vi "DB UI - Transaction Details.vi"(7 "DB Connection":T4={"Open"=TRUE, "Close"=TRUE}, 8 "error in (no error)":errorcluster, 10 "Transaction":T5, 11 "connection reference 2":T2) -> (0 "SUMMARY":errorcluster, 3 "connection reference":T2)   [LabVIEW 2013]
uses:
  <vilib>/addons/database/Connection.llb/Conn ObjectReference.ctl
  Controls/DB - OpenClose.ctl
  Controls/Transaction Cluster.ctl
  Controls/Debug Tab.ctl
  <vilib>/Utility/miscctls.llb/LVPointTypeDef.ctl
  <vilib>/addons/database/Connection.llb/Conn Execute.vi
  <vilib>/addons/database/Recordset.llb/Rec Fetch Recordset Data (R).vi
  <vilib>/addons/database/Recordset.llb/Rec Destroy - Connection.vi
  Controls/Global SRTRS.vi
  <vilib>/addons/database/Connection.llb/DB Tools Open Connec (String).vi
  <vilib>/addons/database/_DB Variant To Data/Database Variant To Data.xnode
  <vilib>/addons/database/NI_Database_API.lvlib
panel:
  in  "Tab Control":T1
  out "Connection Information":T3={"Connection "="SQL Server 32bit HPEnvy", "Username"="admin", "Password"="admin123"}
  in  "DB.Schema.Table\nSRTRS.Execute.Header":string="SRTRS.Execute.Header"
  in  "DB.Schema.Table \nSRTRS.Config.Plant":string="SRTRS.Config.Plant"
  out "data":string[](array[string])
  out "SQL Statement":string
  in  "DB.Schema.Table \nSRTRS.Config.Station":string="SRTRS.Config.Station"
  in  "DB.Schema.Table \nSRTRS.Execute.TransactionResult":string="SRTRS.Execute.TransactionResult"
  in  "DB.Schema.Table \nSRTRS.Config.System":string="SRTRS.Config.System"
  out "Close 2":errorcluster
  in  "Details [CaptionOnly]":string caption="Details"
  in  "Header [CaptionOnly]":string caption="Header"
  in  "Close":bool caption="Setup Save"
  out "[PerformedOn]":string caption="Performed On"
  out "[LastSavedOn]":string caption="Last Saved On"
  out "[LastSavedBy]":string caption="Last Saved By"
  out "Station [Description]":string caption="Station"
  out "System [Description]":string caption="System"
  out "Plant [Description]":string caption="Plant"
  out "[StationId]":string caption="Station"
  out "[SystemId]":string caption="System"
  out "[PlantId]":string caption="Plant"
  out "[TransactionRunNo]":string caption="Run No."
  out "[TransactionNo]":string caption="Transaction No."
  # "2014-10-28 13:44\nh.[PlantId]                          ,p.[Description]           ,h.[StationId]                  ,st.[Description]             ,sy.[SystemId]                ,sy.[Description]           ,h.[LastSavedBy]           ,h.[LastSavedOn]          ,t.[PerformedOn]"
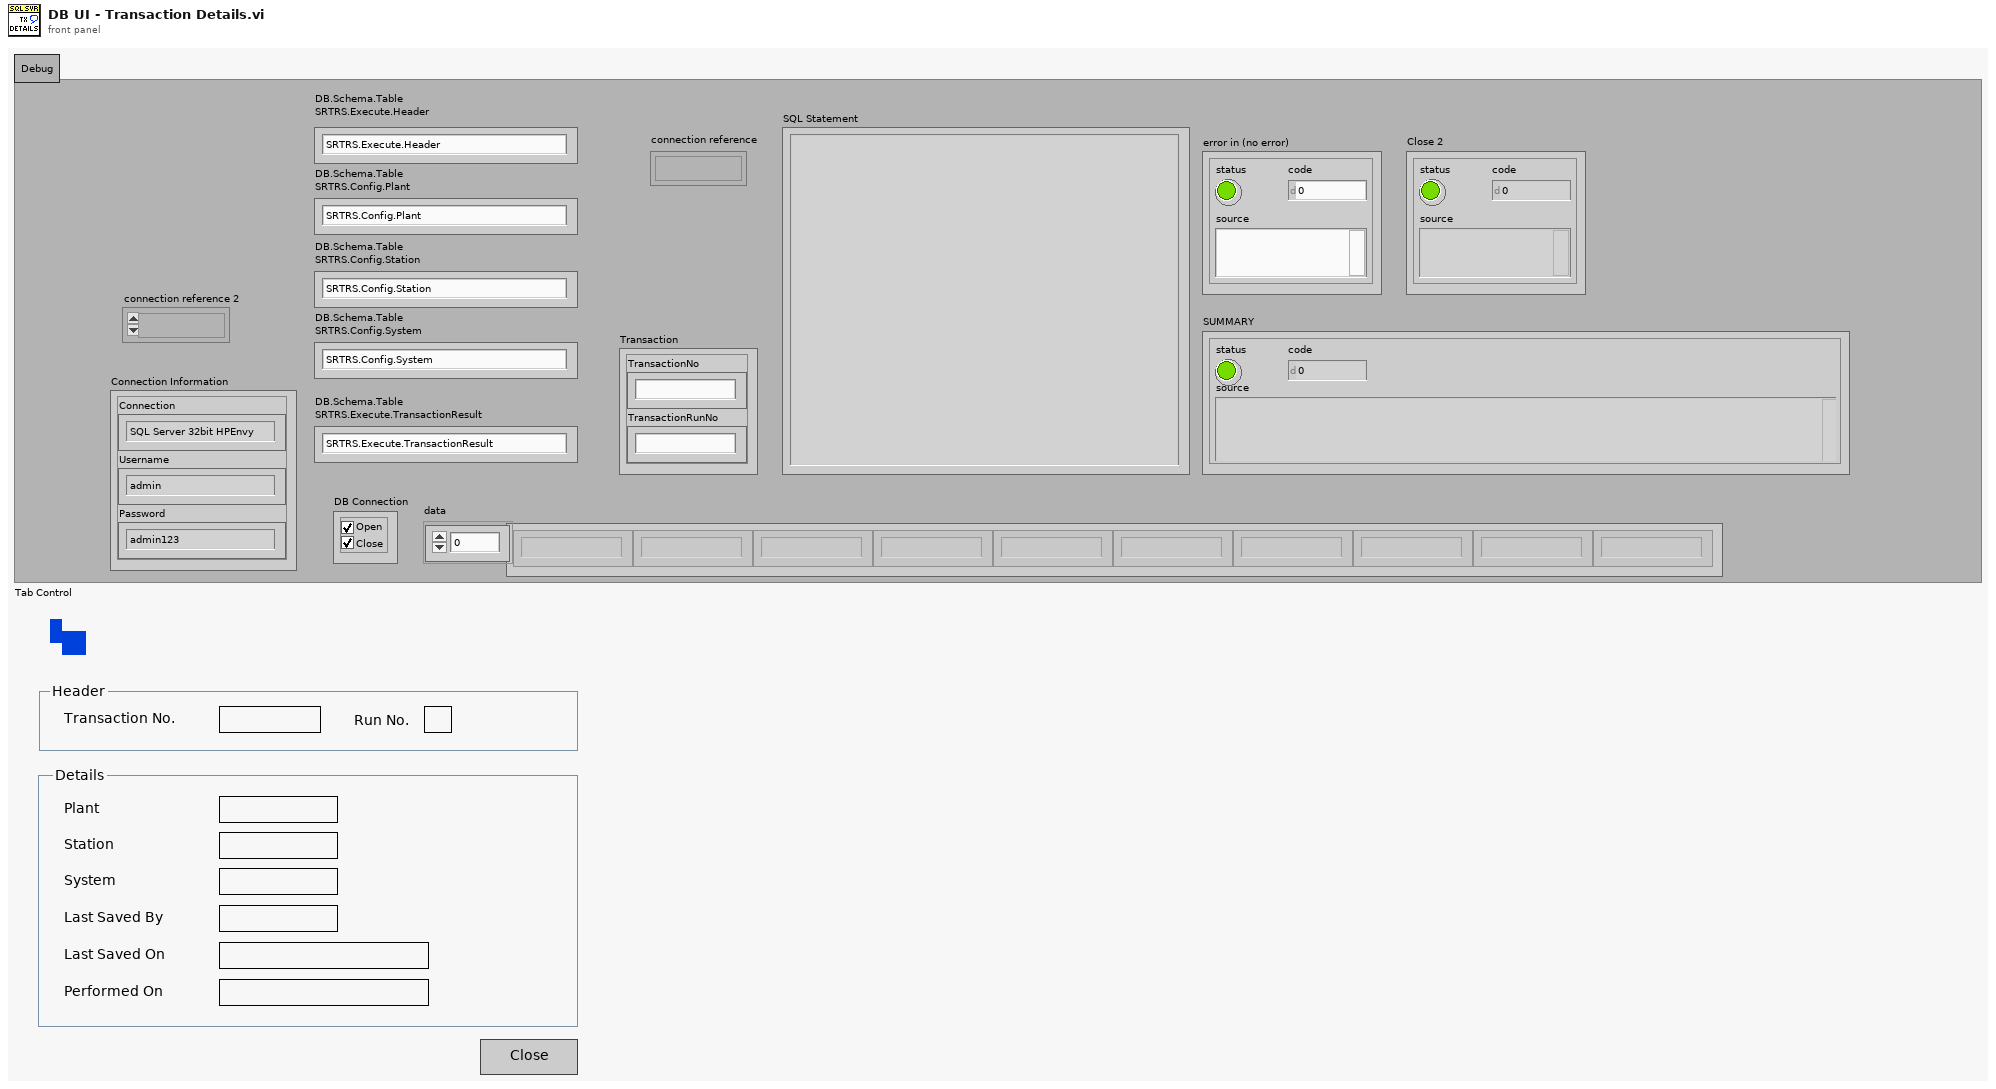
[diagram p1: front panel]
types:
  T1 = typedef "Debug Tab.ctl" = enum32{"Debug"}
  T2 = typedef "NI_Database_API.lvlib/Conn ObjectReference.ctl" = refnum<k1>
  T3 = cluster{"Connection ":string, "Username":string, "Password":string}
  T4 = typedef "DB - OpenClose.ctl" = cluster{"Open":bool, "Close":bool}
  T5 = typedef "Transaction Cluster.ctl" = cluster{"TransactionNo":string, "TransactionRunNo":string}
  T6 = typedef "LVPointTypeDef.ctl" = cluster{"Horizontal":i16, "Vertical":i16}
  T7 = typedef "Enum - InteractiveMode-SubVIMode.ctl" = enum16{"Interactive", "subVI Mode"}
  T8 = typedef "DB - DB.Schema.Table.ctl" = cluster{"DB":string, "Schema":string, "Table":string}
  T9 = typedef "Connection Information Cluster.ctl" = cluster{"Connection ":string, "Username":string, "Password":string}
  T10 = typedef "NI_Database_API.lvlib/Rec ObjectReference.ctl" = refnum<k1>
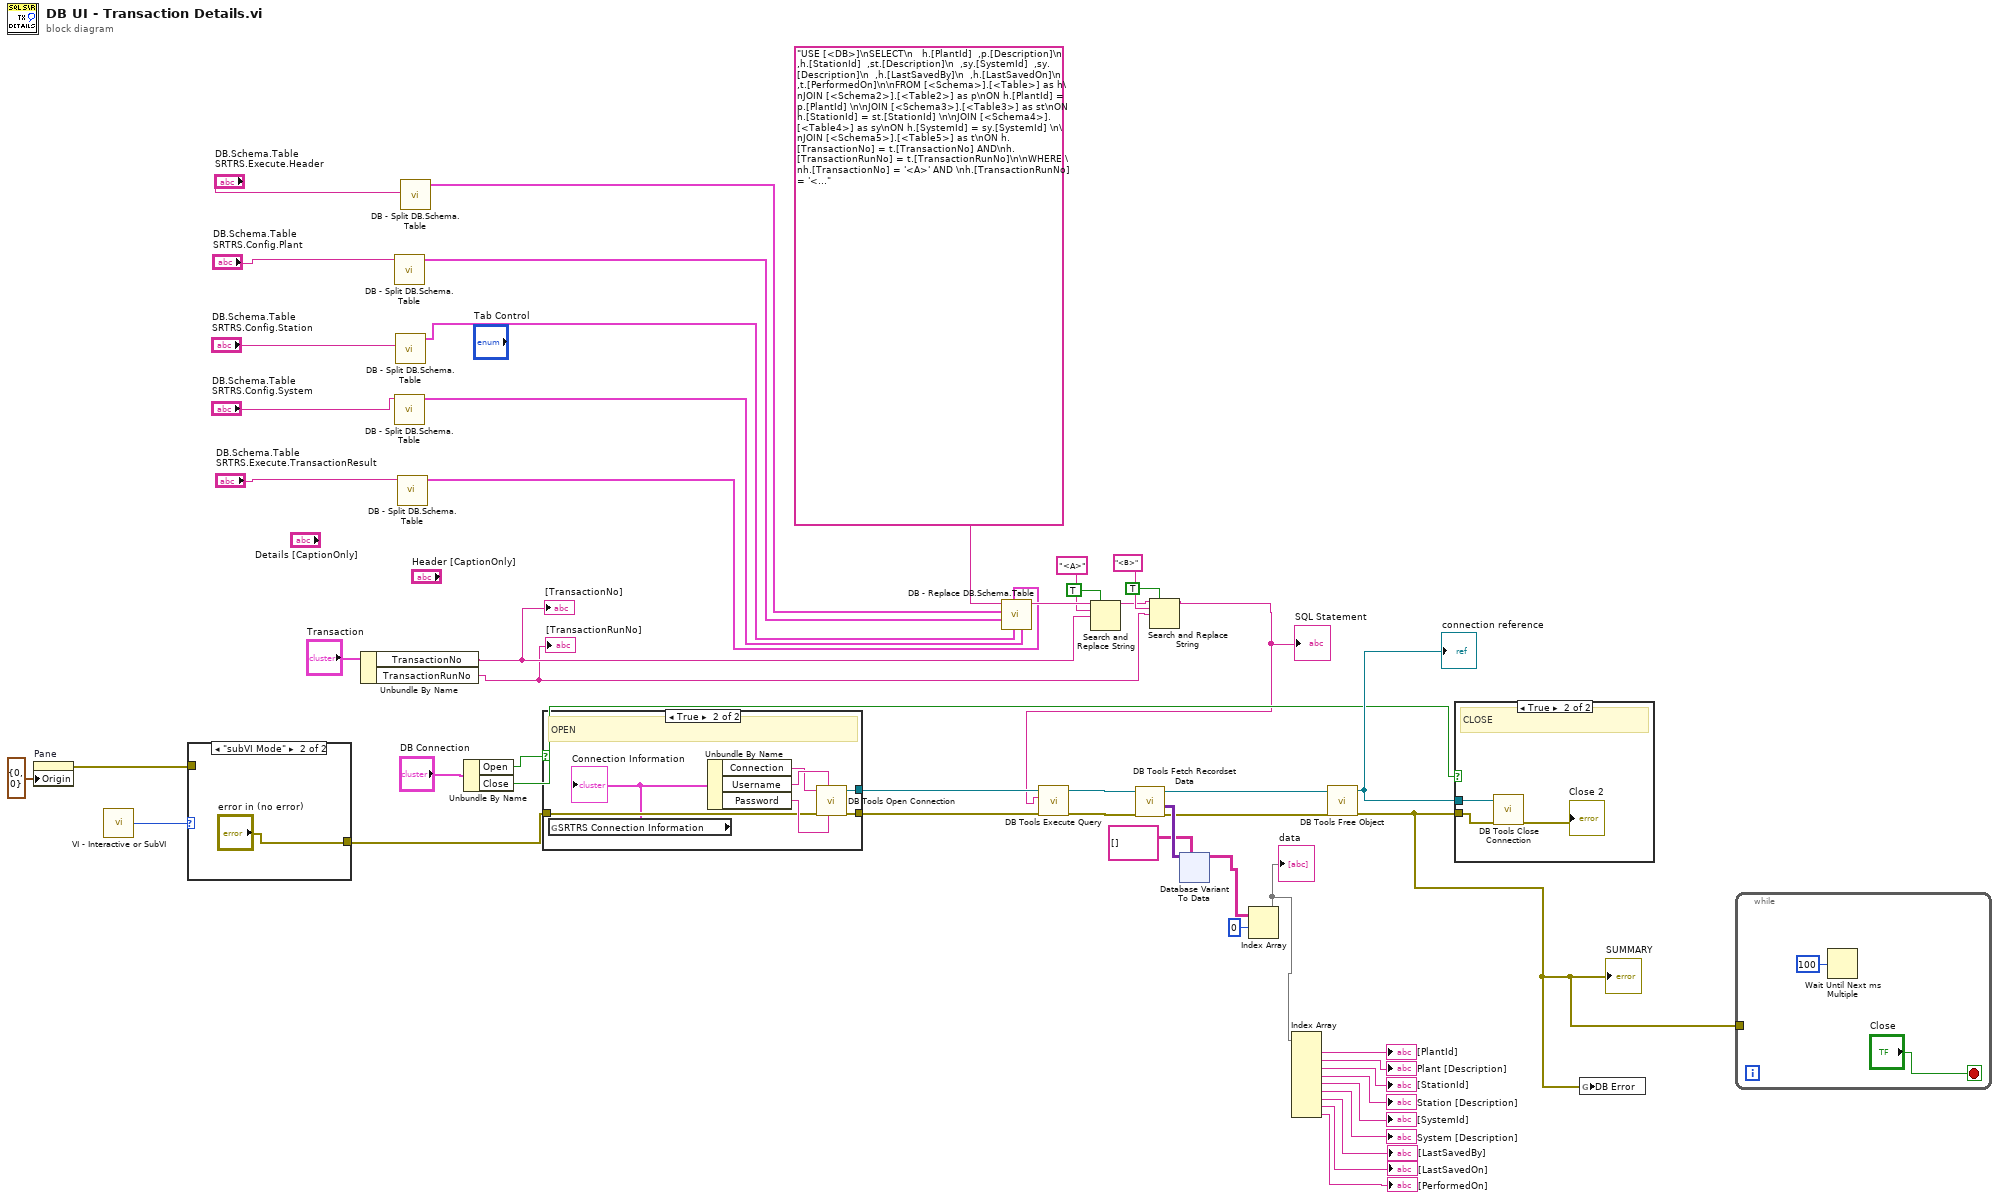
[diagram p0: block diagram]
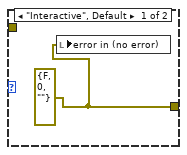
[diagram p3: hidden frame]
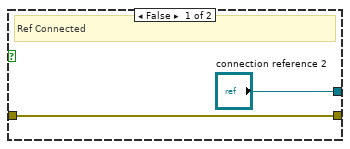
[diagram p4: hidden frame]
diagram:
  n1 = property on="Pane" class="Pane"("Origin"=T6 {"Horizontal"=0, "Vertical"=0}) -> (error out=w20:errorcluster)  [unwired: 2 in, 1 out]
  n2 = call "VI - Interactive or SubVI.vi"() -> ("Mode"=w48:T7)  [unwired: 5 in]
  n3 = case shown="\"subVI Mode\"" w48 {
    tunnel: [w51 "error in (no error)"] -> w47
    tunnel: w20 -> [_ _]
    frame "Interactive", Default {
      w51 = errorcluster {"status"=FALSE, "code"=0, "source"=""} ("error in (no error)")
      n4 = local write "error in (no error)"(w51) -> ()
    }
    frame "subVI Mode" {
    }
  }
  n5 = Unbundle By Name("Transaction") -> ("TransactionNo"=w13:string, "TransactionRunNo"=w12:string)
  "[TransactionNo]" <- w13
  "[TransactionRunNo]" <- w12
  n6 = call "DB - Split DB.Schema.Table.vi"("DB.Schema.Table"="DB.Schema.Table \nSRTRS.Config.Plant") -> ("DB.Schema.Table"=w30:T8)  [unwired: 10 in]
  n7 = call "DB - Split DB.Schema.Table.vi"("DB.Schema.Table"="DB.Schema.Table \nSRTRS.Config.System") -> ("DB.Schema.Table"=w14:T8)  [unwired: 10 in]
  n8 = call "DB - Split DB.Schema.Table.vi"("DB.Schema.Table"="DB.Schema.Table \nSRTRS.Config.Station") -> ("DB.Schema.Table"=w18:T8)  [unwired: 10 in]
  n9 = call "DB - Split DB.Schema.Table.vi"("DB.Schema.Table"="DB.Schema.Table \nSRTRS.Execute.TransactionResult") -> ("DB.Schema.Table"=w15:T8)  [unwired: 10 in]
  n10 = call "DB - Split DB.Schema.Table.vi"("DB.Schema.Table"="DB.Schema.Table\nSRTRS.Execute.Header") -> ("DB.Schema.Table"=w34:T8)  [unwired: 10 in]
  n11 = Unbundle By Name("DB Connection") -> ("Open"=w49:bool, "Close"=w37:bool)
  n12 = case shown="True" w49 {
    tunnel: ["connection reference 2" w58] -> w40
    tunnel: w47 -> [w53 w57]
    tunnel: [w53 w56] -> w39
    frame False {
      # "Ref Connected"
    }
    frame True {
      # "OPEN"
      n13 = global read "Global SRTRS.vi" "SRTRS Connection Information"() -> (w55:T9)
      "Connection Information" <- w55
      n14 = Unbundle By Name(w55) -> ("Connection"=w60:string, "Username"=w61:string, "Password"=w59:string)
      n15 = call-poly <vilib>:"DB Tools Open Connection.vi"("password"=w59, "userID"=w61, "error in (no error)"=w57, "connection information"=w60) -> ("error out"=w56:errorcluster, "connection reference"=w58:T2)  [unwired: 4 in]
    }
  }
  n16 = call "DB - Replace DB.Schema.Table.vi"("DB.Schema.Table 4"=w14, "DB.Schema.Table 3"=w18, "DB.Schema.Table 5"=w15, "DB.Schema.Table 2"=w30, "DB.Schema.Table"=w34, "string in"="USE [<DB>]\nSELECT\n   h.[PlantId]  ,p.[Description]\n  ,h.[StationId]  ,st.[Description]\n  ,sy.[SystemId]  ,sy.[Description]\n  ,h.[LastSavedBy]\n  ,h.[LastSavedOn]\n  ,t.[PerformedOn]\n\nFROM [<Schema>].[<Table>] as h\nJOIN [<Schema2>].[<Table2>] as p\nON h.[PlantId] = p.[PlantId] \n\nJOIN [<Schema3>].[<Table3>] as st\nON h.[StationId] = st.[StationId] \n\nJOIN [<Schema4>].[<Table4>] as sy\nON h.[SystemId] = sy.[SystemId] \n\nJOIN [<Schema5>].[<Table5>] as t\nON h.[TransactionNo] = t.[TransactionNo] AND\nh.[TransactionRunNo] = t.[TransactionRunNo]\n\nWHERE \nh.[TransactionNo] = '<A>' AND \nh.[TransactionRunNo] = '<B>' AND\nh.[Inactive] = '0' AND \np.[Inactive] = '0' AND \nst.[Inactive] = '0' AND \nsy.[Inactive] = '0' AND \nt.[Inactive] = '0' \n\n") -> ("string out"=w32:string)  [unwired: 4 in, 1 out]
  n17 = Search and Replace String(replace all?=TRUE ("replace all? (F)"), input string=w32, search string="<A>", replace string=w13) -> (result string=w25:string)  [unwired: 4 in, 3 out]
  n18 = Search and Replace String(replace all?=TRUE ("replace all? (F)"), input string=w25, search string="<B>", replace string=w12) -> (result string=w24:string)  [unwired: 4 in, 3 out]
  "SQL Statement" <- w24
  n19 = call-poly <vilib>:"DB Tools Execute Query.vi"("error in (no error)"=w39, "SQL query"=w24, "connection reference"=w40) -> ("error out"=w46:errorcluster, "recordset reference"=w45:T10)  [unwired: 5 in]
  n20 = call-poly <vilib>:"DB Tools Fetch Recordset Data.vi"("error in (no error)"=w46, "recordset reference"=w45) -> ("error out"=w41:errorcluster, "recordset data"=w44:variant[][], "recordset reference out"=w42:T10)  [unwired: 3 in]
  n21 = xnode "Database Variant To Data"("database variant"=w44, "type"=string[][] []) -> ("data"=w23:string[][])  [unwired: 1 in, 1 out]
  n22 = Index Array(array=w23, index (row)=0) -> (element=w11:string[])  [unwired: 1 in]
  "data" <- w11
  n23 = Index Array(array=w11) -> (element #1=→"[PlantId]":string, element #2=→"Plant [Description]":string, element #3=→"[StationId]":string, element #4=→"Station [Description]":string, element #5=→"[SystemId]":string, element #6=→"System [Description]":string, element #7=→"[LastSavedBy]":string, element #8=→"[LastSavedOn]":string, element #9=→"[PerformedOn]":string)  [unwired: 9 in]
  n24 = call-poly <vilib>:"DB Tools Free Object.vi"("error in (no error)"=w41, "recordset reference"=w42) -> ("error out"=w1:errorcluster, "connection reference"=w38:T2)  [unwired: 8 in]
  "SUMMARY" <- w1
  "connection reference" <- w38
  n25 = case shown="True" w37 {
    tunnel: w38 -> [_ w64]
    tunnel: w1 -> [_ w63]
    frame False {
      # "Ref Connected"
    }
    frame True {
      # "CLOSE"
      n26 = call <vilib>:"DB Tools Close Connection.vi"("error in (no error)"=w63, "connection reference"=w64) -> ("error out"=→"Close 2":errorcluster)  [unwired: 5 in]
    }
  }
  n27 = global write "Global SRTRS.vi" "DB Error"(w1) -> ()
  n28 = while {
    tunnel: w1 -> [_]
    stop <- "Close" stop-if-true
    n29 = Wait Until Next ms Multiple(millisecond multiple=u32 100) -> ()  [unwired: 1 out]
  }
